vi "Dashboard Main.vi"() -> ()   [LabVIEW 2016]
uses:
  <vilib>/event_ctls.llb/eventvkey.ctl
  <vilib>/Rock Robotics/WPI/Dashboard/WPI_DashboardLogging Global.vi
  <vilib>/Utility/miscctls.llb/LVRowAndColumnTypeDef.ctl
  <vilib>/Rock Robotics/Network Tables/NT Read Numeric Array.vi
  <vilib>/Rock Robotics/Network Tables/NT Write Boolean.vi
panel:
  in  "Camera Settings Right":T1={"Frame Rate"=30, "Compression"=30, "Size"=1, "DB Camera Config"=FALSE} {"Frame Rate" scale=1.0..30.0; "Compression" scale=100.0..-1.0; "Size" items=["640x480", "320x240", "160x120"]}
  in  "Camera Name Right":string(combo)="No Camera Selection"
  out "Camera Info":cluster{"Mbps LED":bool, "Mbps":dbl, "fps":dbl} {"fps" format="%#.1g"; "Mbps" format="%#.1g"}
  in  "Camera Settings":T1={"Frame Rate"=30, "Compression"=30, "Size"=1, "DB Camera Config"=FALSE} {"Frame Rate" scale=1.0..30.0; "Compression" scale=100.0..-1.0; "Size" items=["640x480", "320x240", "160x120"]}
  in  "TCP":refnum<k5>
  in  "Rec Mode":enum32{"Stop", "Record", "Playback"}(radio)
  out "Robot IP":string
  out "Image Message":string="Timeout in Camera Communications"
  in  "Dashboard Tab":T2(tab)
  in  "Select Auto":string(combo)="Select Autonomous ..."
  out "NT Connection":bool
  out "MotorChart R":cluster{"Numeric":dbl, "Numeric":dbl}(graph)
  out "MotorChart L":cluster{"Numeric":dbl, "Numeric":dbl}(graph)
  out "MotorSliders R":cluster{"MotorSlide1":dbl, "MotorSlide2":dbl} {"MotorSlide2" scale=-1.0..1.0 scale format="%#_2e"; "MotorSlide1" scale=-1.0..1.0 scale format="%#_2e"}
  out "MotorSliders L":cluster{"MotorSlide1":dbl, "MotorSlide2":dbl} {"MotorSlide2" scale=-1.0..1.0 scale format="%#_2e"; "MotorSlide1" scale=-1.0..1.0 scale format="%#_2e"}
  out "Gyro":dbl(knob) scale=0.0..360.0
  out "JS1 Z":dbl(slide) scale=-1.0..1.0 scale format="%#_2e"
  out "JS1 Graph":cluster{"X":dbl, "Y":dbl}[](graph)
  out "JS1 Buttons":T3
  out "JS2 Z":dbl(slide) scale=-1.0..1.0 scale format="%#_2e"
  out "JS2 Graph":cluster{"X":dbl, "Y":dbl}[](graph)
  out "JS2 Buttons":T3
  out "Mode":T4(ring)=enum."Auto Disabled"
  in  "Overdrive Enabled?":bool
  in  "Trim":dbl(slide) scale=0.0..1.0
  out "Sonar":dbl
  out "Camera Image Right":T5(plugin-control)
  in  "DB/String 9":string
  in  "DB/String 8":string
  in  "DB/String 7":string
  in  "DB/String 6":string
  in  "DB/String 5":string
  in  "DB/String 4":string
  in  "DB/String 3":string
  in  "DB/String 2":string
  in  "DB/String 1":string
  in  "DB/String 0":string
  in  "DB/Slider 0":dbl(slide) scale=0.0..1.0
  in  "DB/Slider 1":dbl(slide) scale=0.0..5.0
  in  "DB/Slider 2":dbl(slide) scale=0.0..5.0
  in  "DB/Slider 3":dbl(slide) scale=0.0..5.0
  out "DB/LED 3":bool
  out "DB/LED 2":bool
  out "DB/LED 1":bool
  out "DB/LED 0":bool
  in  "DB/Button 3":bool
  in  "DB/Button 2":bool
  in  "DB/Button 1":bool
  in  "DB/Button 0":bool caption="New Name"
  in  "Scaling factor (V/in)":dbl=0.0098
  out "distance":dbl(slide)=125.0 scale=0.0..250.0 scale format="%3d"
  out "Z Acceleration":dbl
  out "Y Acceleration":dbl
  out "X Acceleration":dbl
  in  "Acc.Stop":bool
  in  "Test Slider":dbl(slide) scale=0.0..100.0 scale format="%#_3g"
  in  "On/Off":bool caption="Solenoid"
  in  "Test Name":u16(ring) items=["Select the test to run..."]
  in  "Test Tree":string(tree)
  in  "Motor":cluster{"Value":dbl, "Enable":bool} {"Value" scale=-1.0..1.0 scale format="%#_3g"}
  out "Progress":T6 {"Test Progress" scale=0.0..100.0}
  in  "Rev/Fwd":cluster{"Forward":bool, "Reverse":bool}
  in  "Test Ring":u16(ring) items=["Monochrome", "Color"]
  out "Cmd Status":string
  in  "Execute Command":bool
  in  "Command Params":string[][](table)
  in  "Command Selection":i32(listbox)
  in  "CheckList":i32(listbox)
  out "Tree":string(tree)
  out "Camera Image":T5(plugin-control)
  in  "Camera Name":string(combo)="No Camera Selection"
  # "HW"
  # "HW"
  # "Joysticks"
  # "Drive Motors"
  # "Front"
  # "Right"
  # "Left"
  # "Back"
  # "This tab is a great place for autonomous settings and robot-specific values.\nPlace controls and indicators inside this tab and match name to\nDashboard Variables on robot. You can also delete this comment."
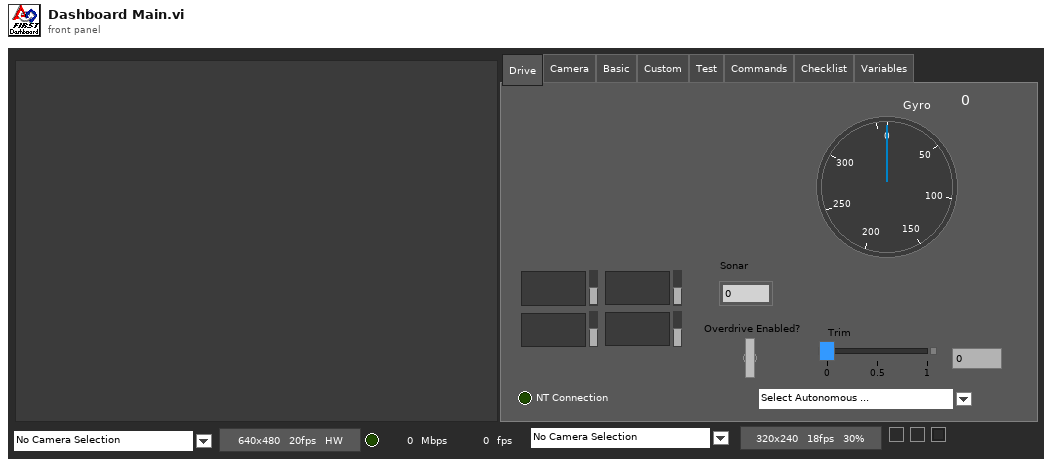
[diagram p1: front panel]
types:
  T1 = cluster{"Frame Rate":i32, "Compression":i32, "Size":u16, "DB Camera Config":bool}
  T2 = enum32{"Drive", "Camera", "Basic", "Custom", "Test", "Commands", "Checklist", "Variables"}
  T3 = cluster{bool, bool, bool, bool, bool, bool, bool, bool, bool, bool, bool, bool}
  T4 = enum8{"Tele-Op Disabled", "Tele-Op Enabled", "Auto Disabled", "Auto Enabled", "Test Disabled", "Test Enabled", "Disconnected", "No Code", "E-Stop"}
  T5 = typedef "IMAQ Image.ctl" = refnum<image>
  T6 = cluster{"Test Progress":u8, "Test Progress Text":string}
  T7 = typedef "Image Type" = u32
  T8 = cluster{"IDs":cluster{"RPC field ID":u16, "Unique ID":u16}, "String":string}
  T9 = enum32{"Drive", "Basic", "Custom", "Test", "Checklist", "Variables"}
  T10 = cluster{"Error Strings":string, "Disable Counts":cluster{u16, u16}, "Rail Faults":cluster{u16, u16, u16}, "Robot IP":string, "DB Mode":u8, "Event Info":cluster{"Name":string, "Type":u8, "Number":u16, "Replay":u8}}
  T11 = cluster{"Storage":cluster{"Disk Free":u64, "RAM Block":u32, "RAM free":u32}, "CPU Utilization":cluster{"CPU % ISR":sgl, "CPU % Time Crit":sgl, "CPU % Timed Str":sgl, "CPU % High":sgl, "CPU % Above":sgl, "CPU % Normal":sgl, "CPU % Low":sgl}, "CAN":cluster{"% Bus Utilization":sgl, "Bus Off Cnt":u32, "TX_FIFO Full Cnt":u32, "Receive Error Cnt":u8, "Transmit Error Cnt":u8}, "HID":cluster{"HID Outputs":u32, "Rumble Low":u16, "Rumble High":u16}[]}
  T12 = cluster{"Status bits":cluster{"Test Mode":bool, "Autonomous":bool, "Enabled":bool, "Code Start":bool, "Brownout":bool, "Reserved 2":bool, "Reserved 3":bool, "E-Stop":bool}, "Code Trace":cluster{"Disabled":bool, "TeleOp":bool, "Auto":bool, "Test":bool}, "Controller Type":enum16{"unknown", "cRIO", "roboRio"}, "Code?":enum16{"unknown", "noCode", "code"}, "Battery V":dbl}
  T13 = cluster{"Control Bits":cluster{"TestMode":bool, "Autonomous":bool, "Enabled":bool, "FMS Present":bool, bool, bool, bool, "E-Stop":bool}, "Team Station ":u8, "Countdown":sgl, "Joystick Values":cluster{"Axes":dbl[], "Buttons":bool[], "POVs":i16[]}[]}
  T14 = cluster{"Axes":dbl[], "Buttons":bool[], "POVs":i16[]}[]
  T15 = cluster{"Axes":dbl[], "Buttons":bool[], "POVs":i16[]}
  T16 = cluster{"Buttons[0]":bool, "Buttons[1]":bool, "Buttons[2]":bool, "Buttons[3]":bool, "Buttons[4]":bool, "Buttons[5]":bool, "Buttons[6]":bool, "Buttons[7]":bool, "Buttons[8]":bool, "Buttons[9]":bool, "Buttons[10]":bool, "Buttons[11]":bool}
  T17 = cluster{"Camera Image":refnum<vi>, "Dashboard Tab":refnum<vi>, void, "Rec Mode":refnum<vi>, "Test Slider":refnum<vi>, "On/Off ":refnum<vi>, "Test Ring":refnum<vi>, "Rev/Fwd":refnum<vi>, "Test Name":refnum<vi>, "Motor":refnum<vi>, "Progress":refnum<vi>, "CheckList":refnum<vi>, "Tree":refnum<vi>, "Test Tree":refnum<vi>, "Command Params":refnum<vi>, "Command Selection":refnum<vi>, "Execute Command":refnum<vi>, "Cmd Status":refnum<vi>, "Camera Settings":refnum<vi>, "Camera Name":refnum<vi>, "Camera Info":refnum<vi>, "Camera Settings Right":refnum<vi>, "Camera Name Right":refnum<vi>, "Camera Image Right":refnum<vi>}
  T18 = cluster{"Operation":enum16{"Update", "Clear"}, "Color Box":u32}[]
  T19 = typedef "eventvkey.ctl" = enum16{"ASCII", "Enter", "Return", "Shift", "Ctrl", "Alt", "Cmd", "Opt", "Caps", "NumLock", "Clear", "Break", "Up", "Down", "Left", "Right", "Insert", "Delete", "Home", "End", "PageUp", "PageDown", "Escape", "Help", "Pause", "ScrollLock", "F1", "F2", "F3", "F4", "F5", "F6", "F7", "F8", "F9", "F10", "F11", "F12", "F13", "F14", "F15", "F16", "F17", "F18", "F19", "F20", "F21", "F22", "F23", "F24", "Play", "VolumeUp", "VolumeDown", "Mute", "Two Byte Char"}
  T20 = cluster{"Image Size":bool, "Image Type":bool, "Pixel Value":bool, "ROI Information":bool, "Zoom Factor":bool}
  T21 = cluster{"Operation":enum16{"Update", "Clear"}, "Color Box":u32}
  T22 = typedef "LVRowAndColumnTypeDef.ctl" = cluster{"Row":i32, "Column":i32}
  T23 = cluster{"Shift":bool, "Ctrl":bool, "Alt":bool, "Cmd":bool, "Opt":bool}
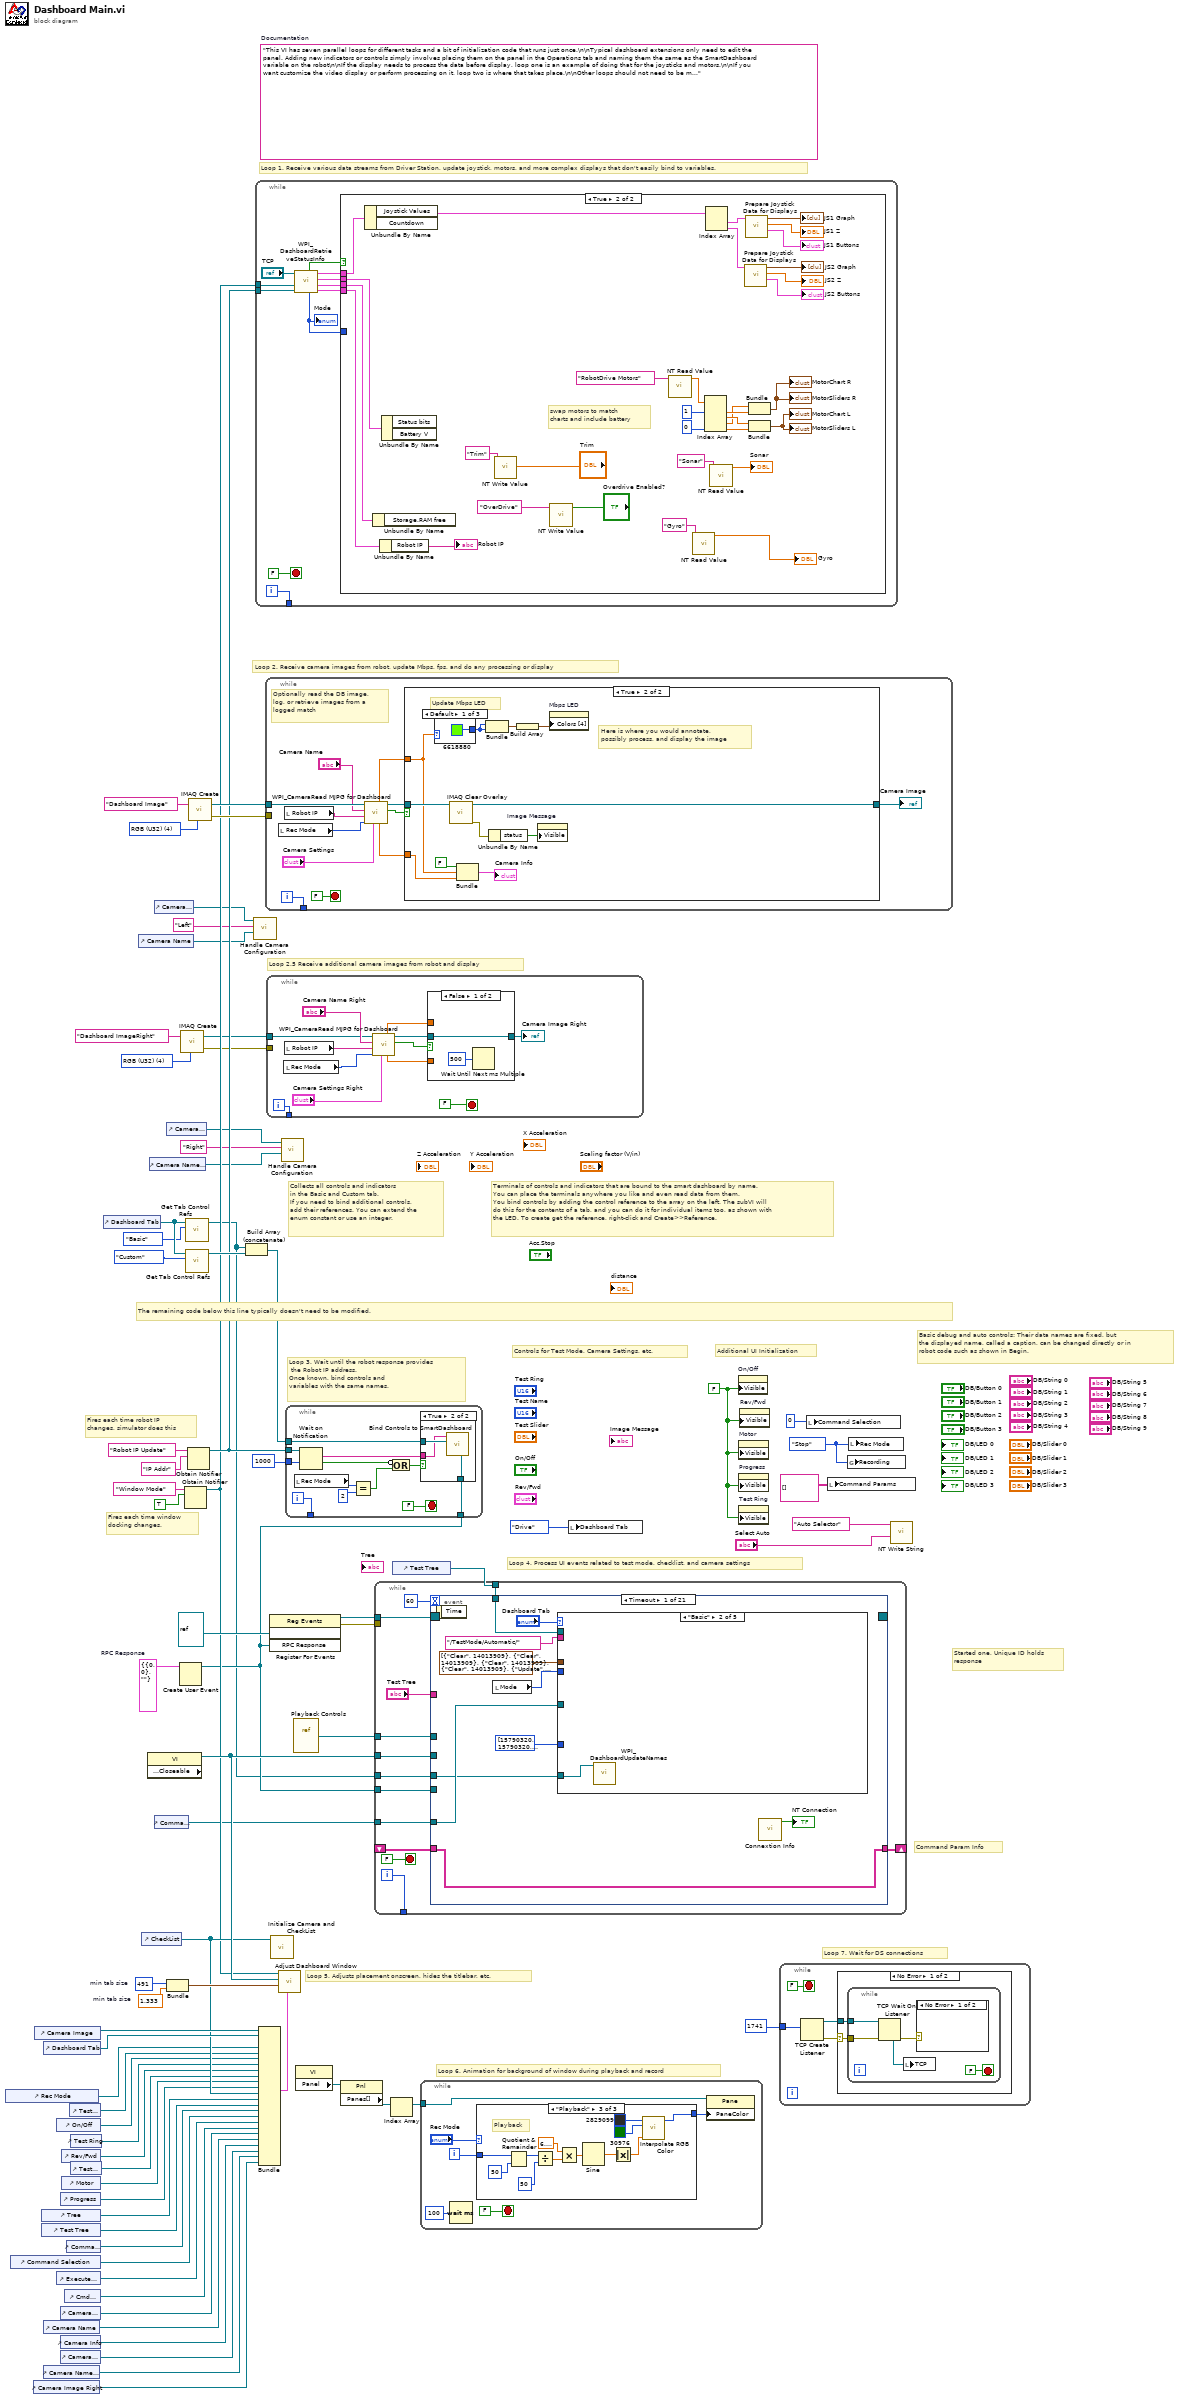
[diagram p0: block diagram]
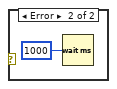
[diagram p3: hidden frame]
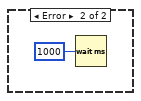
[diagram p4: hidden frame]
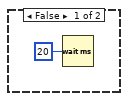
[diagram p5: hidden frame]
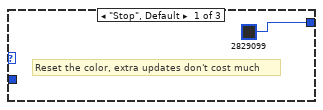
[diagram p6: hidden frame]
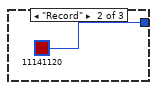
[diagram p7: hidden frame]
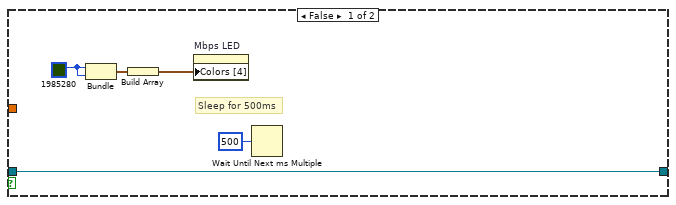
[diagram p9: hidden frame]
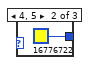
[diagram p10: hidden frame]
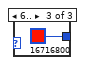
[diagram p11: hidden frame]
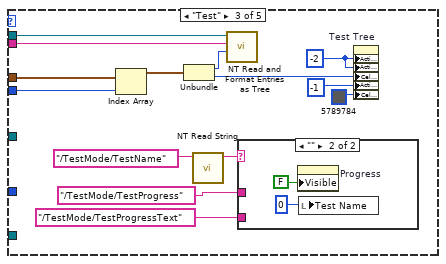
[diagram p13: hidden frame]
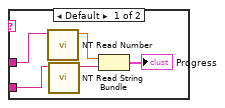
[diagram p14: hidden frame]
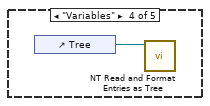
[diagram p15: hidden frame]
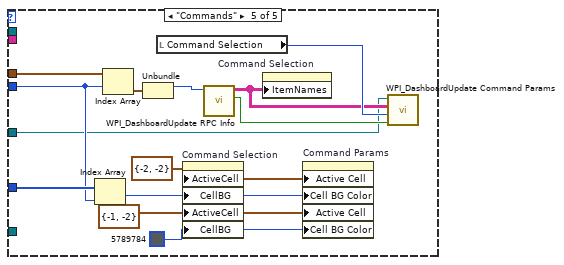
[diagram p16: hidden frame]
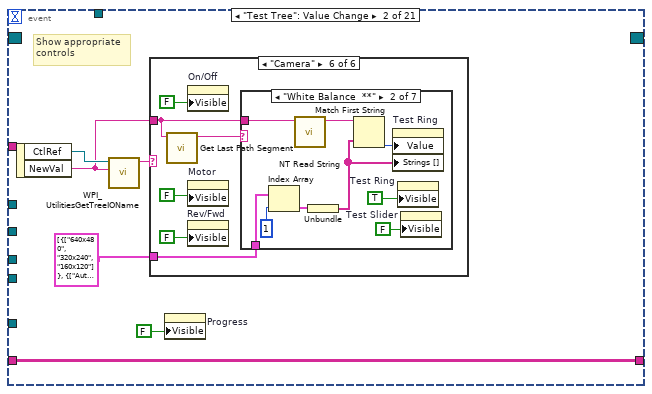
[diagram p17: hidden frame]
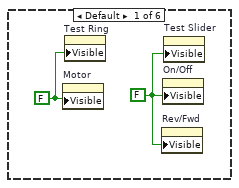
[diagram p18: hidden frame]
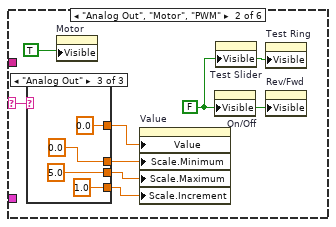
[diagram p19: hidden frame]
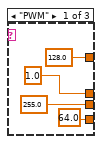
[diagram p20: hidden frame]
diagram:
  w11 = T7 4 items=["Grayscale (U8)", "Grayscale (I16)", "Grayscale (SGL)", "Complex (CSG)", "RGB (U32)", "HSL (U32)", "RGB (U64)"] ("Image Type")
  w27 = T8 {"IDs"={"RPC field ID"=0, "Unique ID"=0}, "String"=""}  # RPC Response
  w50 = 491  # min tab size
  w49 = 1.333  # min tab size
  w57 = enum32{"Stop", "Record", "Playback"}."Stop" ("Rec Mode")
  w34 = FALSE ("Visible")
  (unwired) "This VI has seven parallel loops for different tasks and a bit of initialization code that runs just once.\n\nTypical dashboard extensions only need to edit the panel. Adding new indicators or controls simply involves placing them on the panel in the Operations tab and naming them the same as the SmartDashboard variable on the robot\n\nIf the display needs to process the data before display, loop one is an example of doing that for the joysticks and motors.\n\nIf you want customize the video display or perform processing on it, loop two is where that takes place.\n\nOther loops should not need to be modified. They are pretty standard, and document the task they perform."  # Documentation
  w74 = T7 4 items=["Grayscale (U8)", "Grayscale (I16)", "Grayscale (SGL)", "Complex (CSG)", "RGB (U32)", "HSL (U32)", "RGB (U64)"] ("Image Type")
  # "Loop 2.5 Receive additional camera images from robot and display"
  # "Command Param Info"
  # "Started one, Unique ID holds\nresponse"
  # "Loop 7. Wait for DS connections"
  # "Basic debug and auto controls: Their data names are fixed, but\nthe displayed name, called a caption, can be changed directly or in\nrobot code such as shown in Begin."
  # "Controls for Test Mode, Camera Settings, etc."
  # "Additional UI Initialization"
  # "Loop 6. Animation for background of window during playback and record"
  # "Fires each time robot IP\nchanges, simulator does this"
  # "Fires each time window\ndocking changes."
  # "Collects all controls and indicators\nin the Basic and Custom tab.\nIf you need to bind additional controls,\nadd their references. You can extend the\nenum constant or use an integer."
  # "The remaining code below this line typically doesn't need to be modified."
  # "Loop 4. Process UI events related to test mode, checklist, and camera settings"
  # "Terminals of controls and indicators that are bound to the smart dashboard by name.\nYou can place the terminals anywhere you like and even read data from them.\nYou bind controls by adding the control reference to the array on the left. The subVI will\ndo this for the contents of a tab, and you can do it for individual items too, as shown with\nthe LED. To create get the reference, right-click and Create>>Reference."
  # "Loop 3. Wait until the robot response provides\n the Robot IP address.\nOnce known, bind controls and\nvariables with the same names."
  # "Loop 5. Adjusts placement onscreen, hides the titlebar, etc."
  # "Loop 1. Receive various data streams from Driver Station, update joystick, motors, and more complex displays that don't easily bind to variables."
  # "Loop 2. Receive camera images from robot, update Mbps, fps, and do any processing or display"
  n1 = control-ref of="Rec Mode"() -> (w40:refnum<vi>)
  n2 = control-ref of="Command Selection"() -> (w26:refnum<vi>)
  n3 = control-ref of="Camera Image Right"() -> (w2:refnum<vi>)
  n4 = control-ref of="Camera Image"() -> (w52:refnum<vi>)
  n5 = control-ref of="Tree"() -> (w44:refnum<vi>)
  n6 = control-ref of="Test Tree"() -> (w43:refnum<vi>)
  n7 = control-ref of="Dashboard Tab"() -> (w51:refnum<vi>)
  n8 = control-ref of="Camera Name"() -> (w17:refnum<vi>)
  n9 = control-ref of="Camera Name Right"() -> (w3:refnum<vi>)
  n10 = control-ref of="Execute Command"() -> (w28:refnum<vi>)
  n11 = control-ref of="On/Off"() -> (w38:refnum<vi>)
  n12 = control-ref of="Progress"() -> (w35:refnum<vi>)
  n13 = control-ref of="Camera Settings"() -> (w18:refnum<vi>)
  n14 = control-ref of="Camera Info"() -> (w16:refnum<vi>)
  n15 = control-ref of="Camera Settings Right"() -> (w4:refnum<vi>)
  n16 = control-ref of="Rev/Fwd"() -> (w36:refnum<vi>)
  n17 = control-ref of="Motor"() -> (w41:refnum<vi>)
  n18 = control-ref of="Cmd Status"() -> (w22:refnum<vi>)
  n19 = control-ref of="Command Params"() -> (w29:refnum<vi>)
  n20 = control-ref of="Test Slider"() -> (w39:refnum<vi>)
  n21 = control-ref of="Test Ring"() -> (w37:refnum<vi>)
  n22 = control-ref of="Test Name"() -> (w42:refnum<vi>)
  n23 = control-ref of="Dashboard Tab"() -> (w55:refnum<vi>)
  n24 = control-ref of="Camera Name"() -> (w19:refnum<vi>)
  n25 = control-ref of="CheckList"() -> (w45:refnum<vi>)
  n26 = property class="VI" props=["Front Panel.Closeable"]() -> (reference out=w56:refnum<vi>)  [unwired: 2 in, 2 out]
  n27 = control-ref of="Camera Name Right"() -> (w7:refnum<vi>)
  n28 = control-ref of="Camera Settings"() -> (w20:refnum<vi>)
  n29 = control-ref of="Command Params"() -> (w21:refnum<vi>)
  n30 = control-ref of="Camera Settings Right"() -> (w8:refnum<vi>)
  n31 = Bundle("min tab size"=w50, "min tab size"=w49) -> (w48:cluster{"min tab size":i32, "min tab size":dbl})  [unwired: 1 in]
  n32 = Create User Event(user event datatype=w27) -> (user event=w23:refnum<user-event>)  [unwired: 1 in, 1 out]
  n33 = call "IMAQ Create"("Image Name"="Dashboard ImageRight", "Image Type"=w11) -> ("New Image"=w10:T5, "error out"=w9:errorcluster)  [unwired: 2 in, 1 out]
  n34 = Obtain Notifier(name (unnamed)="Window Mode", notification data type=TRUE) -> (notifier out=w32:refnum<notifier>)  [unwired: 2 in, 2 out]
  n35 = call <vilib>:"Get Tab Control Refs.vi"("Page Index"=T9."Basic" ("Dashboard Tab"), "TabControl in"=w55) -> ("ControlsOnPage"=w15:refnum<vi>[])  [unwired: 9 in]
  n36 = call <vilib>:"Get Tab Control Refs.vi"("Page Index"=T9."Custom" ("Dashboard Tab"), "TabControl in"=w55) -> ("ControlsOnPage"=w54:refnum<vi>[])  [unwired: 9 in]
  n37 = Obtain Notifier(name (unnamed)="Robot IP Update", notification data type="IP Addr" ("name (unnamed)")) -> (notifier out=w33:refnum<notifier>)  [unwired: 2 in, 2 out]
  n38 = call "IMAQ Create"("Image Name"="Dashboard Image", "Image Type"=w74) -> ("New Image"=w72:T5, "error out"=w71:errorcluster)  [unwired: 2 in, 1 out]
  n39 = Build Array (concatenate)(w15, w54) -> (w53:refnum<vi>[])
  n40 = call "Handle Camera Configuration.vi"("CameraNameRef"=w19, "Camera File Name"="Left", "ClusterRef"=w20) -> ()  [unwired: 9 in]
  n41 = while {
    tunnel: [w84] -> _
    tunnel: w33 -> [w78]
    tunnel: w32 -> [w75]
    i -> [w84]
    stop <- FALSE stop-if-true
    n42 = call <vilib>:"WPI_DashboardRetrieveStatusInfo.vi"("Binding Refnum"=w78, "Window Mode Notifier"=w75, "TCP Cnx"="TCP") -> ("Power and Errors"=w79:T10, "Robot Metrics"=w82:T11, "Status Info"=w83:T12, "Control Info"=w80:T13, "Robot Mode"=w77:T4, "Process?"=w81:bool)  [unwired: 3 in]
    "Mode" <- w77
    n43 = case shown="True" w81 {
      tunnel: w83 -> [_ w118]
      tunnel: w82 -> [_ w117]
      tunnel: w80 -> [_ w116]
      tunnel: w79 -> [_ w115]
      tunnel: w77 -> [_ _]
      frame False {
        n44 = Wait (ms)(milliseconds to wait=u32 20) -> ()  [unwired: 1 out]
      }
      frame True {
        # "swap motors to match\ncharts and include battery"
        n45 = Unbundle By Name(w116) -> ("Joystick Values"=w106:T14)  [unwired: 1 out]
        n46 = Unbundle By Name(w117) -> ()  [unwired: 1 out]
        n47 = Unbundle By Name(w115) -> ("Robot IP"=→"Robot IP":string)
        n48 = Unbundle By Name(w118) -> ()  [unwired: 2 out]
        n49 = call-poly <vilib>:"NT Write Value.vi"("Numeric"="Trim", "Name"="Trim") -> ()  [unwired: 9 in, 1 out]
        n50 = call-poly <vilib>:"NT Write Value.vi"("Boolean"="Overdrive Enabled?", "Name"="OverDrive") -> ()  [unwired: 9 in, 1 out]
        n51 = call-poly <vilib>:"NT Read Value.vi"("Name"="RobotDrive Motors") -> ("Numeric Array"=w96:dbl[])  [unwired: 9 in, 1 out]
        n52 = call-poly <vilib>:"NT Read Value.vi"("Name"="Gyro") -> ("Numeric"=→"Gyro":dbl)  [unwired: 9 in, 1 out]
        n53 = Index Array(array=w96, index #1=1, index #4=0) -> (element #1=w110:dbl, element #2=w111:dbl, element #3=w109:dbl, element #4=w114:dbl)  [unwired: 2 in]
        n54 = Index Array(array=w106) -> (element #1=w105:T15, element #2=w101:T15)  [unwired: 2 in]
        n55 = call-poly <vilib>:"NT Read Value.vi"("Name"="Sonar") -> ("Numeric"=→"Sonar":dbl)  [unwired: 9 in, 1 out]
        n56 = call "Prepare Joystick Data for Displays.vi"("Joystick Values"=w101) -> ("Buttons"=→"JS2 Buttons":T16, "Z Axis"=→"JS2 Z":dbl, "Cartesian Data"=→"JS2 Graph":cluster{"X axis":dbl, "X axis":dbl}[])  [unwired: 8 in]
        n57 = call "Prepare Joystick Data for Displays.vi"("Joystick Values"=w105) -> ("Buttons"=→"JS1 Buttons":T16, "Z Axis"=→"JS1 Z":dbl, "Cartesian Data"=→"JS1 Graph":cluster{"X axis":dbl, "X axis":dbl}[])  [unwired: 8 in]
        n58 = Bundle("Numeric"=w109, "Numeric"=w110) -> (→"MotorChart R" →"MotorSliders R":cluster{"Numeric":dbl, "Numeric":dbl})  [unwired: 1 in]
        n59 = Bundle("Numeric"=w111, "Numeric"=w114) -> (→"MotorChart L" →"MotorSliders L":cluster{"Numeric":dbl, "Numeric":dbl})  [unwired: 1 in]
      }
    }
  }
  n60 = Bundle("Camera Image"=w52, "Dashboard Tab"=w51, "Rec Mode"=w40, "Test Slider"=w39, "On/Off"=w38, "Test Ring"=w37, "Rev/Fwd"=w36, "Test Name"=w42, "Motor"=w41, "Progress"=w35, "CheckList"=w45, "Tree"=w44, "Test Tree"=w43, "Command Params"=w29, "Command Selection"=w26, "Execute Command"=w28, "Cmd Status"=w22, "Camera Settings"=w18, "Camera Name"=w17, "Camera Info"=w16, "Camera Settings Right"=w4, "Camera Name Right"=w3, "Camera Image Right"=w2) -> (w1:T17)  [unwired: 2 in]
  n61 = while {
    tunnel: w72 -> [w128]
    tunnel: w71 -> [_]
    tunnel: [w129] -> _
    i -> [w129]
    stop <- FALSE stop-if-true
    # "Optionally read the DB image,\nlog, or retrieve images from a\nlogged match"
    n62 = local read "Rec Mode"() -> (w124:enum32{"Stop", "Record", "Playback"})
    n63 = local read "Robot IP"() -> (w123:string)
    n64 = call <vilib>:"WPI_CameraRead MJPG for Dashboard.vi"("Camera Settings"="Camera Settings", "Rec Mode"=w124, "Robot IP"=w123, "Camera Name"="Camera Name", "Refnum in"=w128) -> ("Active"=w126:bool, "Refnum out"=w127:T5, "FPS"=w125:dbl, "Bandwidth (Mbps)"=w122:dbl)  [unwired: 3 in]
    n65 = case shown="True" w126 {
      tunnel: w127 -> [w131 w142]
      tunnel: w122 -> [_ w139]
      tunnel: w125 -> [_ w140]
      tunnel: [w131 w136] -> w119
      frame False {
        w133 = u32 1985280 ("Color Box")
        # "Sleep for 500ms"
        n66 = Bundle("Color Box"=w133, "Color Box"=w133) -> (w134:cluster{"Color Box":u32, "Color Box":u32})  [unwired: 1 out]
        n67 = Build Array(w134) -> (w132:cluster{"Color Box":u32, "Color Box":u32}[])
        n68 = property on="Mbps LED" class="Bool (strict)"("Colors [4]"=w132) -> ()  [unwired: 2 in, 2 out]
        n69 = Wait Until Next ms Multiple(millisecond multiple=u32 500) -> ()  [unwired: 1 out]
      }
      frame True {
        # "Here is where you would annotate,\npossibly process, and display the image"
        # "Update Mbps LED"
        n70 = case shown="Default" w139 {
          tunnel: [u32 6618880 ("Color Box") u32 16776722 ("Color Box") u32 16716800 ("Color Box")] -> w143
          frame Default {
          }
          frame 4, 5 {
          }
          frame 6.. {
          }
        }
        n71 = call "IMAQ Clear Overlay"("Image"=w142) -> ("error out"=w145:errorcluster, "Image Out"=w136:T5)  [unwired: 2 in, 7 out]
        n72 = Bundle(FALSE, "Bandwidth (Mbps)"=w139, "FPS"=w140) -> (→"Camera Info":cluster{bool, "Bandwidth (Mbps)":dbl, "FPS":dbl})  [unwired: 1 in]
        n73 = Bundle("Color Box"=w143, "Color Box"=w143) -> (w144:cluster{"Color Box":u32, "Color Box":u32})  [unwired: 1 out]
        n74 = Unbundle By Name(w145) -> ("status"=w146:bool)
        n75 = Build Array(w144) -> (w141:cluster{"Color Box":u32, "Color Box":u32}[])
        n76 = property on="Image Message" class="Str"("Visible"=w146) -> ()  [unwired: 2 in, 2 out]
        n77 = property on="Mbps LED" class="Bool (strict)"("Colors [4]"=w141) -> ()  [unwired: 2 in, 2 out]
      }
    }
    "Camera Image" <- w119
  }
  n78 = while {
    tunnel: w10 -> [w160]
    tunnel: w9 -> [_]
    tunnel: [w154] -> _
    i -> [w154]
    stop <- FALSE stop-if-true
    n79 = local read "Rec Mode"() -> (w158:enum32{"Stop", "Record", "Playback"})
    n80 = local read "Robot IP"() -> (w159:string)
    n81 = call <vilib>:"WPI_CameraRead MJPG for Dashboard.vi"("Camera Settings"="Camera Settings Right", "Rec Mode"=w158, "Robot IP"=w159, "Camera Name"="Camera Name Right", "Refnum in"=w160) -> ("Active"=w153:bool, "Refnum out"=w156:T5, "FPS"=w151:dbl, "Bandwidth (Mbps)"=w152:dbl)  [unwired: 3 in]
    n82 = case shown="False" w153 {
      tunnel: w156 -> [w162 w164]
      tunnel: w152 -> [_ _]
      tunnel: w151 -> [_ _]
      tunnel: [w162 w164] -> w150
      frame False {
        n83 = Wait Until Next ms Multiple(millisecond multiple=u32 500) -> ()  [unwired: 1 out]
      }
      frame True {
      }
    }
    "Camera Image Right" <- w150
  }
  n84 = register-events(refnum<vi> refnum, w23) -> (reference out=w61:refnum<event-registration>, error out=w60:errorcluster)  [unwired: 2 in]
  n85 = call "Initialize Camera and CheckList.vi"("ListBox in"=w45) -> ()  [unwired: 11 in]
  n86 = call "Adjust Dashboard Window.vi"("Sizing Refnums"=w1, "Size Constraints"=w48, "VI"=w56, "WIn Mode"=w32) -> ()  [unwired: 8 in]
  n87 = call "Handle Camera Configuration.vi"("CameraNameRef"=w7, "Camera File Name"="Right", "ClusterRef"=w8) -> ()  [unwired: 9 in]
  n88 = while {
    tunnel: w53 -> [w176]
    tunnel: w33 -> [w174]
    tunnel: [w172] -> _
    tunnel: u32 1000 ("milliseconds to wait") -> [w171]
    tunnel: w23 -> [w165]
    i -> [w172]
    stop <- FALSE stop-if-true
    n89 = local read "Rec Mode"() -> (w167:enum32{"Stop", "Record", "Playback"})
    n90 = Wait on Notification(notifier=w174, timeout in ms (-1)=w171) -> (notification=w173:string, timed out?=w169:bool)  [unwired: 2 in, 2 out]
    n91 = Equal?(x=w167, y=u16 2 ("Rec Mode")) -> (x = y?=w168:bool)
    n92 = Compound Arithmetic op=OR(invert w169, w168) -> (w170:bool)
    n93 = case shown="True" w170 {
      tunnel: w176 -> [_ w179]
      tunnel: w173 -> [_ w178]
      tunnel: w165 -> [_ w177]
      frame False {
      }
      frame True {
        n94 = call <vilib>:"Bind Controls to SmartDashboard.vi"("RPC ref"=w177, "Bound Control Refs"=w179, "Server IP Address"=w178) -> ()  [unwired: 9 in]
      }
    }
  }
  n95 = vi-ref "Playback Controls.vi"() -> (w62:refnum<vi>)
  n96 = property class="VI"() -> ("Panel"=w64:refnum<vi>)  [unwired: 2 in, 2 out]
  n97 = property class="Pnl"(reference=w64) -> ("Panes[]"=w65:refnum<vi>[])  [unwired: 1 in, 2 out]
  n98 = Index Array(array=w65) -> (element=w63:refnum<vi>)  [unwired: 1 in]
  n99 = control-ref of="Test Tree"() -> (w66:refnum<vi>)
  n100 = while {
    tunnel: [w189] -> _
    tunnel: w66 -> [w188]
    tunnel: w62 -> [w187]
    tunnel: w61 -> [w186]
    tunnel: w60 -> [_]
    tunnel: w56 -> [w185]
    tunnel: w23 -> [w184]
    tunnel: w21 -> [w183]
    shift-right: [w182] -> _
    shift-left: _ -> [w181]
    tunnel: w15 -> [w180]
    i -> [w189]
    stop <- FALSE stop-if-true
    n101 = event shown="[0] Timeout" {
      selector: w186 -> [_ _ _ _ _ _ _ _ _ _ _ _ _ _ _ _ _ _ _ _ _]
      dyn-events: [_ _ _ _ _ _ _ _ _ _ _ _ _ _ _ _ w445 _ _ _ _] -> _
      timeout: u32 60 ("milliseconds to wait") -> [_ _ _ _ _ _ _ _ _ _ _ _ _ _ _ _ _ _ _ _ _]
      tunnel: w188 -> [w201 _ _ _ _ _ _ _ _ _ _ _ _ _ _ _ _ _ _ _ _]
      tunnel: "Test Tree" -> [_ _ _ _ _ _ _ _ _ _ _ w412 w420 w422 w426 w434 _ _ _ _ _]
      tunnel: w187 -> [_ _ _ _ _ _ _ _ _ _ _ _ _ _ _ _ w447 _ w465 _ _]
      tunnel: w185 -> [_ _ _ _ _ _ _ _ _ _ _ _ _ _ _ _ w443 _ _ _ _]
      tunnel: w184 -> [_ _ _ _ _ _ _ _ _ _ _ _ _ _ _ _ w439 _ _ _ _]
      tunnel: w183 -> [w196 _ _ _ _ _ w363 _ _ _ _ _ _ _ _ _ _ _ _ _ _]
      tunnel: [w195 w240 w342 w347 w356 w360 w361 w370 w380 w387 w399 w411 w418 w421 w425 w433 w438 w460 w462 w466 w477] -> w182
      tunnel: w181 -> [w195 w240 w342 w347 w356 w360 w361 _ _ w387 w399 w411 w418 w421 w425 w433 w438 w460 w462 w466 w477]
      tunnel: w180 -> [w193 _ _ _ _ _ _ _ _ _ _ _ _ _ _ _ _ _ _ _ _]
      event Timeout {
        n102 = event-data() -> ()  [unwired: 1 in, 1 out]
        n103 = local read "Mode"() -> (w198:T4)
        n104 = case shown="\"Basic\"" "Dashboard Tab" {
          tunnel: w201 -> [_ _ w217 _ _]
          tunnel: "/TestMode/Automatic/" ("Name Pattern") -> [_ _ w216 _ _]
          tunnel: T18 [{"Operation"=enum."Clear", "Color Box"=14013909}, {"Operation"=enum."Clear", "Color Box"=14013909}, {"Operation"=enum."Clear", "Color Box"=14013909}, {"Operation"=enum."Clear", "Color Box"=14013909}, {"Operation"=enum."Update", "Color Box"=14013909}, {"Operation"=enum."Update", "Color Box"=16777215}, {"Operation"=enum."Clear", "Color Box"=14013909}, {"Operation"=enum."Clear", "Color Box"=14013909}, {"Operation"=enum."Clear", "Color Box"=14013909}] -> [_ _ w209 _ w233]
          tunnel: w198 -> [_ _ w208 _ w232]
          tunnel: u32[] [15790320, 15790320, 15790320, 15790320, 16777215, 16777215, 15790320, 15790320, 15790320] -> [_ _ _ _ w238]
          tunnel: w196 -> [_ _ _ _ w226]
          tunnel: w193 -> [_ w203 _ _ _]
          frame "Custom", Default {
          }
          frame "Basic" {
            n105 = call <vilib>:"WPI_DashboardUpdateNames.vi"("Controls on Tab"=w203) -> ()  [unwired: 11 in]
          }
          frame "Test" {
            w215 = -2 ("Active Item:Row Number")
            n106 = Index Array(array=w209, index=w208) -> (element=w210:T21)
            n107 = Unbundle(w210) -> ("Operation"=w211:enum16{"Update", "Clear"}, "Color Box"=w212:u32)
            n108 = call <vilib>:"NT Read String.vi"("Name"="/TestMode/TestName") -> ("String"=w206:string)  [unwired: 9 in, 1 out]
            n109 = call <vilib>:"NT Read and Format Entries as Tree.vi"("Operation"=w211, "Name Pattern"=w216, "Tree Refnum"=w217) -> ()  [unwired: 7 in, 2 out]
            n110 = case shown="\"\"" w206 {
              tunnel: "/TestMode/TestProgress" ("Name") -> [w219 _]
              tunnel: "/TestMode/TestProgressText" ("Name") -> [w218 _]
              frame Default {
                n111 = call <vilib>:"NT Read Number.vi"("Name"=w219) -> ("Numeric"=w220:dbl)  [unwired: 9 in, 1 out]
                n112 = call <vilib>:"NT Read String.vi"("Name"=w218) -> ("String"=w221:string)  [unwired: 9 in, 1 out]
                n113 = Bundle("Numeric"=w220, "String"=w221) -> (→"Progress":cluster{"Numeric":dbl, "String":string})  [unwired: 1 in]
              }
              frame "" {
                n114 = property on="Progress" class="Clust (strict)"("Visible"=FALSE) -> ()  [unwired: 2 in, 2 out]
                n115 = local write "Test Name"(u16 0) -> ()
              }
            }
            n116 = property on="Test Tree" class="Tree (strict)"("Active Item Row Number"=w215, "ActiveColNum"=w215, "CellBG"=w212, "Active Item Row Number"=-1 ("Active Item:Row Number"), "CellBG"=u32 5789784 ("Color Box")) -> ()  [unwired: 2 in, 2 out]
          }
          frame "Variables" {
            n117 = control-ref of="Tree"() -> (w225:refnum<vi>)
            n118 = call <vilib>:"NT Read and Format Entries as Tree.vi"("Tree Refnum"=w225) -> ()  [unwired: 9 in, 2 out]
          }
          frame "Commands" {
            w234 = u32 5789784 ("Color Box")
            w235 = T22 {"Row"=-1, "Column"=-2} ("Active Cell:Active Cell")
            w237 = T22 {"Row"=-2, "Column"=-2} ("Active Cell:Active Cell")
            n119 = Index Array(array=w238, index=w232) -> (element=w236:u32)
            n120 = Index Array(array=w233, index=w232) -> (element=w231:T21)
            n121 = Unbundle(w231) -> ("Operation"=w230:enum16{"Update", "Clear"})  [unwired: 1 out]
            n122 = local read "Command Selection"() -> (w229:i32)
            n123 = property on="Command Selection" class="MCListbox (strict)"("ActiveCell"=w237, "CellBG"=w236, "ActiveCell"=w235, "CellBG"=w234) -> ()  [unwired: 2 in, 2 out]
            n124 = call <vilib>:"WPI_DashboardUpdate RPC Info.vi"("Operation"=w230) -> ("update"=w228:bool, "commands"=w227:string[][])  [unwired: 9 in]
            n125 = property on="Command Selection" class="MCListbox (strict)"("ItemNames"=w227) -> ()  [unwired: 2 in, 2 out]
            n126 = property on="Command Params" class="Tbl (strict)"("Active Cell"=w237, "Cell BG Color"=w236, "Active Cell"=w235, "Cell BG Color"=w234) -> ()  [unwired: 2 in, 2 out]
            n127 = call <vilib>:"WPI_DashboardUpdate Command Params.vi"("Update"=w228, "NewVal"=w229, "Commands"=w227, "Param Tbl"=w226) -> ()  [unwired: 7 in, 1 out]
          }
        }
        n128 = call <vilib>:"Connextion Info.vi"() -> ("Connected"=→"NT Connection":bool)  [unwired: 10 in, 1 out]
      }
      event "Test Tree": Value Change {
        # "Show appropriate\ncontrols"
        n129 = event-data() -> ("CtlRef"=w243:refnum<vi>, "NewVal"=w241:string)  [unwired: 1 in]
        n130 = call <vilib>:"WPI_UtilitiesGetTreeIOName.vi"("NewVal"=w241, "TreeControl in"=w243) -> ("I/O Name"=w244:string)  [unwired: 9 in]
        n131 = case shown="\"Camera\"" w244 {
          selector: w244 -> [_ w251 _ w273 w282 _]
          tunnel: w241 -> [_ _ w270 w272 _ w289]
          tunnel: cluster{string[]}[] [{["640x480", "320x240", "160x120"]}, {["Auto", "Fixed indoor", "Fixed outdoor 1", "Fixed outdoor 2", "Fixed fluorescent 1", "Fixed fluorescent 2", "Hold current"]}, {["Auto", "Flicker-free 50 Hz", "Flicker-free 60 Hz", "Hold current"]}, {["None", "Prioritize frame rate", "Prioritize image quality"]}, {["Monochrome", "Color"]}] -> [_ _ _ _ _ w288]
          frame Default {
            w246 = FALSE ("Visible")
            w245 = FALSE ("Visible")
            n132 = property on="Motor" class="Clust (strict)"("Visible"=w245) -> ()  [unwired: 2 in, 2 out]
            n133 = property on="Test Ring" class="Ring (strict)"("Visible"=w245) -> ()  [unwired: 2 in, 2 out]
            n134 = property on="Rev/Fwd" class="Clust (strict)"("Visible"=w246) -> ()  [unwired: 2 in, 2 out]
            n135 = property on="On/Off" class="Bool (strict)"("Visible"=w246) -> ()  [unwired: 2 in, 2 out]
            n136 = property on="Test Slider" class="Slide (strict)"("Visible"=w246) -> ()  [unwired: 2 in, 2 out]
          }
          frame "Analog Out", "Motor", "PWM" {
            w252 = FALSE ("Visible")
            n137 = case shown="\"Analog Out\"" w251 {
              tunnel: [1.0 ("Value") -1.0 ("Value") 0.0 ("Value")] -> w250
              tunnel: [255.0 ("Value") 1.0 ("Value") 5.0 ("Value")] -> w249
              tunnel: [128.0 ("Value") 0.0 ("Value") 0.0 ("Value")] -> w248
              tunnel: [64.0 ("Value") 0.5 ("Value") 1.0 ("Value")] -> w247
              frame "PWM" {
              }
              frame "Motor", Default {
              }
              frame "Analog Out" {
              }
            }
            n138 = property on="Motor" class="Clust (strict)"("Visible"=TRUE) -> ()  [unwired: 2 in, 2 out]
            n139 = property on="Value" class="Slide (strict)"("Value"=w248, "Scale.Minimum"=w250, "Scale.Maximum"=w249, "Scale.Increment"=w247) -> ()  [unwired: 2 in, 2 out]
            n140 = property on="On/Off" class="Bool (strict)"("Visible"=w252) -> ()  [unwired: 2 in, 2 out]
            n141 = property on="Test Slider" class="Slide (strict)"("Visible"=w252) -> ()  [unwired: 2 in, 2 out]
            n142 = property on="Test Ring" class="Ring (strict)"("Visible"=w252) -> ()  [unwired: 2 in, 2 out]
            n143 = property on="Rev/Fwd" class="Clust (strict)"("Visible"=w252) -> ()  [unwired: 2 in, 2 out]
          }
          frame "Servo" {
            w268 = FALSE ("Visible")
            n144 = call <vilib>:"NT Read Number.vi"("Name"=w270) -> ("Numeric"=w269:dbl)  [unwired: 9 in, 1 out]
            n145 = property on="Test Slider" class="Slide (strict)"("Visible"=TRUE, "Scale.Maximum"=170.0 ("Scale.Range:Maximum")) -> ()  [unwired: 2 in, 2 out]
            n146 = local write "Test Slider"(w269) -> ()
            n147 = property on="Motor" class="Clust (strict)"("Visible"=w268) -> ()  [unwired: 2 in, 2 out]
            n148 = property on="Rev/Fwd" class="Clust (strict)"("Visible"=w268) -> ()  [unwired: 2 in, 2 out]
            n149 = property on="On/Off" class="Bool (strict)"("Visible"=w268) -> ()  [unwired: 2 in, 2 out]
            n150 = property on="Test Ring" class="Ring (strict)"("Visible"=w268) -> ()  [unwired: 2 in, 2 out]
          }
          frame "Relay", "Solenoid" {
            w271 = FALSE ("Visible")
            n151 = property on="Motor" class="Clust (strict)"("Visible"=w271) -> ()  [unwired: 2 in, 2 out]
            n152 = property on="Test Slider" class="Slide (strict)"("Visible"=w271) -> ()  [unwired: 2 in, 2 out]
            n153 = Search and Replace String(input string=w272, search string="/Value  **", replace string="/Direction") -> (result string=w278:string)  [unwired: 5 in, 3 out]
            n154 = property on="Test Ring" class="Ring (strict)"("Visible"=w271) -> ()  [unwired: 2 in, 2 out]
            n155 = call <vilib>:"NT Read String.vi"("Name"=w278) -> ("String"=w276:string)  [unwired: 9 in, 1 out]
            n156 = Equal?(x="Both directions", y=w276) -> (x = y?=w274:bool)
            n157 = Not(x=w274) -> (.not. x?=w275:bool)
            n158 = property on="Rev/Fwd" class="Clust (strict)"("Visible"=w274) -> ()  [unwired: 2 in, 2 out]
            n159 = property on="On/Off" class="Bool (strict)"("Visible"=w275, "Caption.Text"=w273) -> ()  [unwired: 2 in, 2 out]
          }
          frame "Compressor", "Digital Out" {
            w281 = FALSE ("Visible")
            # "Get direction and finish"
            n160 = property on="Motor" class="Clust (strict)"("Visible"=w281) -> ()  [unwired: 2 in, 2 out]
            n161 = property on="Test Slider" class="Slide (strict)"("Visible"=w281) -> ()  [unwired: 2 in, 2 out]
            n162 = property on="Test Ring" class="Ring (strict)"("Visible"=w281) -> ()  [unwired: 2 in, 2 out]
            n163 = property on="On/Off" class="Bool (strict)"("Visible"=TRUE, "Caption.Text"=w282) -> ()  [unwired: 2 in, 2 out]
            n164 = property on="Rev/Fwd" class="Clust (strict)"("Visible"=FALSE) -> ()  [unwired: 2 in, 2 out]
          }
          frame "Camera" {
            n165 = call <vilib>:"Get Last Path Segment.vi"("String in"=w289) -> ("String out"=w290:string)  [unwired: 10 in]
            n166 = property on="On/Off" class="Bool (strict)"("Visible"=FALSE) -> ()  [unwired: 2 in, 2 out]
            n167 = property on="Motor" class="Clust (strict)"("Visible"=FALSE) -> ()  [unwired: 2 in, 2 out]
            n168 = property on="Rev/Fwd" class="Clust (strict)"("Visible"=FALSE) -> ()  [unwired: 2 in, 2 out]
            n169 = case shown="\"White Balance  **\"" w290 {
              tunnel: w289 -> [w296 w305 w314 w323 w332 _ w338]
              tunnel: w288 -> [w294 w302 w311 w320 w329 _ _]
              frame "Size  **" {
                n170 = Index Array(array=w294) -> (element=w293:cluster{string[]})  [unwired: 1 in]
                n171 = call <vilib>:"NT Read String.vi"("Name"=w296) -> ("String"=w295:string)  [unwired: 9 in, 1 out]
                n172 = Unbundle(w293) -> (w291:string[])
                n173 = Match First String(2:w291, 3:w295) -> (0:w292:i32)  [unwired: 1 out]
                n174 = property on="Test Ring" class="Ring (strict)"("Value"=w292, "Strings []"=w291) -> ()  [unwired: 2 in, 2 out]
                n175 = property on="Test Ring" class="Ring (strict)"("Visible"=TRUE) -> ()  [unwired: 2 in, 2 out]
                n176 = property on="Test Slider" class="Slide (strict)"("Visible"=FALSE) -> ()  [unwired: 2 in, 2 out]
              }
              frame "White Balance  **" {
                n177 = Index Array(array=w302, index=1) -> (element=w303:cluster{string[]})
                n178 = call <vilib>:"NT Read String.vi"("Name"=w305) -> ("String"=w304:string)  [unwired: 9 in, 1 out]
                n179 = Unbundle(w303) -> (w300:string[])
                n180 = Match First String(2:w300, 3:w304) -> (0:w299:i32)  [unwired: 1 out]
                n181 = property on="Test Ring" class="Ring (strict)"("Value"=w299, "Strings []"=w300) -> ()  [unwired: 2 in, 2 out]
                n182 = property on="Test Ring" class="Ring (strict)"("Visible"=TRUE) -> ()  [unwired: 2 in, 2 out]
                n183 = property on="Test Slider" class="Slide (strict)"("Visible"=FALSE) -> ()  [unwired: 2 in, 2 out]
              }
              frame "Exposure  **" {
                n184 = Index Array(array=w311, index=2) -> (element=w312:cluster{string[]})
                n185 = call <vilib>:"NT Read String.vi"("Name"=w314) -> ("String"=w313:string)  [unwired: 9 in, 1 out]
                n186 = Unbundle(w312) -> (w308:string[])
                n187 = Match First String(2:w308, 3:w313) -> (0:w309:i32)  [unwired: 1 out]
                n188 = property on="Test Ring" class="Ring (strict)"("Value"=w309, "Strings []"=w308) -> ()  [unwired: 2 in, 2 out]
                n189 = property on="Test Ring" class="Ring (strict)"("Visible"=TRUE) -> ()  [unwired: 2 in, 2 out]
                n190 = property on="Test Slider" class="Slide (strict)"("Visible"=FALSE) -> ()  [unwired: 2 in, 2 out]
              }
              frame "Exposure Priority  **" {
                n191 = Index Array(array=w320, index=3) -> (element=w321:cluster{string[]})
                n192 = call <vilib>:"NT Read String.vi"("Name"=w323) -> ("String"=w322:string)  [unwired: 9 in, 1 out]
                n193 = Unbundle(w321) -> (w317:string[])
                n194 = Match First String(2:w317, 3:w322) -> (0:w318:i32)  [unwired: 1 out]
                n195 = property on="Test Ring" class="Ring (strict)"("Value"=w318, "Strings []"=w317) -> ()  [unwired: 2 in, 2 out]
                n196 = property on="Test Ring" class="Ring (strict)"("Visible"=TRUE) -> ()  [unwired: 2 in, 2 out]
                n197 = property on="Test Slider" class="Slide (strict)"("Visible"=FALSE) -> ()  [unwired: 2 in, 2 out]
              }
              frame "Color Enable  **" {
                n198 = Index Array(array=w329, index=4) -> (element=w330:cluster{string[]})
                n199 = call <vilib>:"NT Read String.vi"("Name"=w332) -> ("String"=w331:string)  [unwired: 9 in, 1 out]
                n200 = Unbundle(w330) -> (w326:string[])
                n201 = Match First String(2:w326, 3:w331) -> (0:w327:i32)  [unwired: 1 out]
                n202 = property on="Test Ring" class="Ring (strict)"("Value"=w327, "Strings []"=w326) -> ()  [unwired: 2 in, 2 out]
                n203 = property on="Test Ring" class="Ring (strict)"("Visible"=TRUE) -> ()  [unwired: 2 in, 2 out]
                n204 = property on="Test Slider" class="Slide (strict)"("Visible"=FALSE) -> ()  [unwired: 2 in, 2 out]
              }
              frame Default {
                n205 = property on="Test Ring" class="Ring (strict)"("Visible"=FALSE) -> ()  [unwired: 2 in, 2 out]
                n206 = property on="Test Slider" class="Slide (strict)"("Visible"=FALSE) -> ()  [unwired: 2 in, 2 out]
              }
              frame "Brightness  **", "Color Level  **", "Compression  **", "FPS  **", "Sharpness  **" {
                n207 = call <vilib>:"NT Read Number.vi"("Name"=w338) -> ("Numeric"=w337:dbl)  [unwired: 9 in, 1 out]
                n208 = local write "Test Slider"(w337) -> ()
                n209 = property on="Test Slider" class="Slide (strict)"("Visible"=TRUE, "Scale.Maximum"=100.0 ("Scale.Range:Maximum")) -> ()  [unwired: 2 in, 2 out]
                n210 = property on="Test Ring" class="Ring (strict)"("Visible"=FALSE) -> ()  [unwired: 2 in, 2 out]
              }
            }
          }
        }
        n211 = property on="Progress" class="Clust (strict)"("Visible"=FALSE) -> ()  [unwired: 2 in, 2 out]
      }
      event "Test Name": Mouse Enter {
        # "Populate the ring with the list of tests"
        n212 = event-data() -> ()  [unwired: 1 in, 1 out]
        n213 = call <vilib>:"NT Read String Array.vi"("Name"="/TestMode/TestList") -> ("String Array"=w346:string[])  [unwired: 9 in, 1 out]
        n214 = Build Array (concatenate)("Select the test to run...", w346) -> (w345:string[])
        n215 = property on="Test Name" class="Ring (strict)"("Strings []"=w345) -> ()  [unwired: 2 in, 2 out]
      }
      event "Test Name": Value Change {
        w348 = FALSE ("Visible")
        # "Tell the robot the test name to run"
        n216 = event-data() -> ("NewVal"=w352:u16)  [unwired: 1 in]
        n217 = property on="Test Name" class="Ring (strict)"() -> ("Strings []"=w353:string[])  [unwired: 2 in, 2 out]
        n218 = local write "Progress"(T6 {"Test Progress"=0, "Test Progress Text"=""} ("Progress")) -> ()
        n219 = Index Array(array=w353, index=w352) -> (element=w351:string)
        n220 = call <vilib>:"NT Write String.vi"("String"=w351, "Name"="/TestMode/TestName") -> ()  [unwired: 9 in, 1 out]
        n221 = property on="Progress" class="Clust (strict)"("Visible"=TRUE) -> ()  [unwired: 2 in, 2 out]
        n222 = property on="Motor" class="Clust (strict)"("Visible"=w348) -> ()  [unwired: 2 in, 2 out]
        n223 = property on="Test Slider" class="Slide (strict)"("Visible"=w348) -> ()  [unwired: 2 in, 2 out]
        n224 = property on="On/Off" class="Bool (strict)"("Visible"=w348) -> ()  [unwired: 2 in, 2 out]
        n225 = property on="Rev/Fwd" class="Clust (strict)"("Visible"=w348) -> ()  [unwired: 2 in, 2 out]
        n226 = property on="Test Ring" class="Ring (strict)"("Visible"=w348) -> ()  [unwired: 2 in, 2 out]
      }
      event "Select Auto": Mouse Enter {
        # "Populate the combo box with the list of autonomous options"
        n227 = event-data() -> ()  [unwired: 1 in, 1 out]
        n228 = call <vilib>:"NT Read String Array.vi"("Name"="Auto List") -> ("String Array"=w355:string[])  [unwired: 9 in, 1 out]
        n229 = property on="Select Auto" class="CmbBox"("Strings[]"=w355) -> ()  [unwired: 2 in, 2 out]
      }
      event "Select Auto": Value Change {
        # "User modified the Auto Selection. Write to NT variable so robot knows."
        n230 = event-data() -> ("NewVal"=w358:string)  [unwired: 1 in]
        n231 = call <vilib>:"NT Write String.vi"("String"=w358, "Name"="Auto Selector") -> ()  [unwired: 9 in, 1 out]
      }
      event "Command Selection": Value Change {
        # "Get the params and show in table"
        n232 = event-data() -> ("NewVal"=w364:i32)  [unwired: 1 in]
        n233 = property on="Command Selection" class="MCListbox (strict)"() -> ("ItemNames"=w362:string[][])  [unwired: 2 in, 2 out]
        n234 = call <vilib>:"WPI_DashboardUpdate Command Params.vi"("NewVal"=w364, "Commands"=w362, "Param Tbl"=w363) -> ()  [unwired: 8 in, 1 out]
      }
      event "Execute Command": Value Change {
        # "Started one, Unique ID holds\nresponse"
        n235 = event-data() -> ()  [unwired: 1 in, 1 out]
        n236 = property on="Command Selection" class="MCListbox (strict)"() -> ("ItemNames"=w375:string[][])  [unwired: 2 in, 2 out]
        n237 = Index Array(array=w375, index (row)="Command Selection", index (col)=0) -> (element=w373:string)
        n238 = call <vilib>:"Invoke Commands.vi"("Command Params"="Command Params", "Function Name"=w373) -> ("Params"=w369:u8, "Started"=w368:bool)  [unwired: 7 in, 1 out]
        n239 = Array Subset(array="Command Params", length (row)=w369) -> (w370:string[][])  [unwired: 3 in]
        n240 = Select(t="Executing" ("Cmd Status"), s=w368, f="" ("Cmd Status")) -> (s? t:f=→"Cmd Status":string)
      }
      event "Command Selection": Double Click {
        n241 = event-data() -> ("Row"=w383:i32)  [unwired: 1 in]
        n242 = property on="Command Selection" class="MCListbox (strict)"() -> ("ItemNames"=w386:string[][])  [unwired: 2 in, 2 out]
        n243 = local read "Command Params"() -> (w382:string[][])
        n244 = Index Array(array=w386, index (row)=w383, index (col)=0) -> (element=w384:string)
        n245 = call <vilib>:"Invoke Commands.vi"("Command Params"=w382, "Function Name"=w384) -> ("Params"=w381:u8, "Started"=w376:bool)  [unwired: 7 in, 1 out]
        n246 = Array Subset(array=w382, length (row)=w381) -> (w380:string[][])  [unwired: 3 in]
        n247 = Select(t="Executing" ("Cmd Status"), s=w376, f="" ("Cmd Status")) -> (s? t:f=w377:string)
        n248 = local write "Cmd Status"(w377) -> ()
      }
      event "CheckList": Double Click {
        # "Shift clears all"
        # "Update symbols on the listbox"
        n249 = event-data() -> ("PlatMods.Shift"=w388:bool, "Row"=w390:i32)  [unwired: 1 in]
        n250 = case shown="True" w388 {
          tunnel: w390 -> [w394 _]
          tunnel: 1 -> [w393 _]
          frame False {
            n251 = property on="CheckList" class="LstBox (strict)"() -> ("Item Symbols"=w392:i32[])  [unwired: 2 in, 2 out]
            n252 = Replace Array Subset(array=w392, new element=w393, index=w394) -> (w391:i32[])
            n253 = property on="CheckList" class="LstBox (strict)"("Item Symbols"=w391) -> ()  [unwired: 2 in, 2 out]
          }
          frame True {
            w395 = 0 ("Top Row")
            n254 = property on="CheckList" class="LstBox (strict)"() -> ("Number of Rows"=w397:u32)  [unwired: 2 in, 2 out]
            n255 = Initialize Array(0, w397) -> (w396:i32[])
            n256 = property on="CheckList" class="LstBox (strict)"("Top Row"=w395, "Value"=w395, "Item Symbols"=w396) -> ()  [unwired: 2 in, 2 out]
          }
        }
      }
      event "CheckList": Key Down {
        # "Update symbols on the listbox\nLeft and right keys check and uncheck"
        n257 = event-data() -> ("VKey"=w401:T19)  [unwired: 1 in]
        n258 = case shown="\"Left\", \"Right\"" w401 {
          selector: w401 -> [w406 _]
          tunnel: eventvkey."Left" ("VKey") -> [w404 _]
          frame "Left", "Right" {
            n259 = Equal?(x=w404, y=w406) -> (x = y?=w405:bool)
            n260 = Select(t=0, s=w405, f=1) -> (s? t:f=w407:i32)
            n261 = property on="CheckList" class="LstBox (strict)"() -> ("Item Symbols"=w410:i32[])  [unwired: 2 in, 2 out]
            n262 = Replace Array Subset(array=w410, new element=w407, index="CheckList") -> (w409:i32[])
            n263 = property on="CheckList" class="LstBox (strict)"("Item Symbols"=w409) -> ()  [unwired: 2 in, 2 out]
          }
          frame Default {
          }
        }
      }
      event "Motor.Enable": Value Change {
        # "When the test mode otor enable helper is set, update that\ntree row item's value"
        n264 = event-data() -> ("NewVal"=w416:bool)  [unwired: 1 in]
        n265 = Unbundle("Motor") -> ("Value"=w415:dbl)  [unwired: 1 out]
        n266 = Select(t=w415, s=w416, f=0.0) -> (s? t:f=w413:dbl)
        n267 = call <vilib>:"NT Write Number.vi"("Numeric"=w413, "Name"=w412) -> ()  [unwired: 9 in, 1 out]
      }
      event "Test Slider": Value Change {
        # "When the test mode slider helper is set, update that\ntree row item's value"
        n268 = event-data() -> ("NewVal"=w419:dbl)  [unwired: 1 in]
        n269 = call <vilib>:"NT Write Number.vi"("Numeric"=w419, "Name"=w420) -> ()  [unwired: 9 in, 1 out]
      }
      event "On/Off": Value Change {
        # "When the test mode on/off helper value is set, update that\ntree row item's value"
        n270 = event-data() -> ("NewVal"=w424:bool)  [unwired: 1 in]
        n271 = Boolean To (0,1)(Boolean=w424) -> (0, 1=w423:i16)
        n272 = call <vilib>:"NT Write Number.vi"("Numeric"=w423, "Name"=w422) -> ()  [unwired: 9 in, 1 out]
      }
      event "Rev/Fwd": Value Change {
        # "When the test mode helper value for relays is set, update that\ntree row item's value"
        n273 = event-data() -> ("NewVal.Forward"=w432:bool, "NewVal.Reverse"=w431:bool)  [unwired: 1 in]
        n274 = Boolean To (0,1)(Boolean=w432) -> (0, 1=w428:i16)
        n275 = Boolean To (0,1)(Boolean=w431) -> (0, 1=w430:i16)
        n276 = Negate(x=w430) -> (-x=w429:i16)
        n277 = Add(x=w428, y=w429) -> (x+y=w427:i16)
        n278 = call <vilib>:"NT Write Number.vi"("Numeric"=w427, "Name"=w426) -> ()  [unwired: 9 in, 1 out]
      }
      event "Test Ring": Value Change {
        # "When a test mode helper value is selected from the ring,\nset the tree item's variable to the string value"
        n279 = event-data() -> ("NewVal"=w436:u16)  [unwired: 1 in]
        n280 = property on="Test Ring" class="Ring (strict)"() -> ("Strings []"=w437:string[])  [unwired: 2 in, 2 out]
        n281 = Index Array(array=w437, index=w436) -> (element=w435:string)
        n282 = call <vilib>:"NT Write String.vi"("String"=w435, "Name"=w434) -> ()  [unwired: 9 in, 1 out]
      }
      event "Rec Mode": Value Change {
        # "Update globals for recording mode and path to read log from.\nClear when logging and let NetworkTables set path for vision to\nuse."
        n283 = event-data() -> ("NewVal"=w448:enum32{"Stop", "Record", "Playback"})  [unwired: 1 in]
        n284 = global write "WPI_DashboardLogging Global.vi" "Logging Filename"(path "") -> ()
        n285 = global write "WPI_DashboardLogging Global.vi" "Recording"(w448) -> ()
        n286 = case shown="\"Playback\"" w448 {
          tunnel: w447 -> [_ w450 w459]
          tunnel: [_ _ w458] -> w445
          tunnel: [_ _ w457] -> _
          tunnel: w443 -> [_ _ w455]
          tunnel: cluster{i32, i32} {-250, 170} -> [_ _ w454]
          tunnel: [_ _ T20 {"Image Size"=TRUE, "Image Type"=TRUE, "Pixel Value"=TRUE, "ROI Information"=TRUE, "Zoom Factor"=FALSE} ("Image Information Shown:All Elements")] -> w441
          tunnel: [_ _ TRUE ("Zoom Factor")] -> w440
          tunnel: w439 -> [_ _ w451]
          frame Default {
          }
          frame "Stop", "Record" {
            # "Place Window too"
            n287 = invoke class="VI" method="FP.Close"(reference=w450) -> (reference out=w449:refnum<vi>)  [unwired: 2 in, 2 out]
            n288 = invoke class="VI" method="Abort VI"(reference=w449) -> ()  [unwired: 2 in, 3 out]
          }
          frame "Playback" {
            n289 = call "Open Playback Panel.vi"("Offset"=w454, "DB VI Ref"=w455, "Playback in"=w459) -> ("Playback out"=w456:refnum<vi>)  [unwired: 8 in]
            n290 = register-events(w456, w451) -> (reference out=w458:refnum<event-registration>, error out=w457:errorcluster)  [unwired: 2 in]
          }
        }
        n291 = property on="Camera Image" class="ImageControl"("Image Information Shown"=w441, "Image Information Visible"=w440) -> ()  [unwired: 2 in, 2 out]
        n292 = call <vilib>:"WPI_DashboardNT Log FieldName Cache.vi"("Operation"=enum16{"Lookup/Add", "Index", "Clear"}."Clear") -> ()  [unwired: 8 in, 3 out]
      }
      event Panel Close {
        w461 = enum32{"Stop", "Record", "Playback"}."Stop" ("Rec Mode")
        # "Playback window has been closed, abort"
        n293 = event-data() -> ()  [unwired: 1 in, 4 out]
        n294 = local write "Rec Mode"(w461) -> ()
        n295 = global write "WPI_DashboardLogging Global.vi" "Recording"(w461) -> ()
      }
      event Panel Close {
        # "Abort playback window and ourself"
        n296 = event-data() -> ()  [unwired: 1 in, 4 out]
        n297 = invoke class="VI" method="FP.Close"(reference=w465) -> (reference out=w464:refnum<vi>)  [unwired: 2 in, 2 out]
        n298 = invoke class="VI" method="Abort VI"(reference=w464) -> (error out=w463:errorcluster)  [unwired: 2 in, 2 out]
        n299 = invoke class="VI" method="Abort VI"(error in=w463) -> ()  [unwired: 2 in, 3 out]
      }
      event User Event {
        n300 = event-data() -> ("IDs"=w472:cluster{"RPC field ID":u16, "Unique ID":u16}, "String"=w471:string)  [unwired: 1 in]
        n301 = Bundle("IDs"=w472, "String"=w471) -> (w470:T8)  [unwired: 1 in]
        n302 = call <vilib>:"Retrieve RPC Response.vi"("RPC Response"=w470) -> ("Output"=w468:string[][])  [unwired: 10 in]
        n303 = Build Array (concatenate)(w466, w468) -> (w467:string[][])
        n304 = local write "Command Params"(w467) -> ()
        n305 = local write "Cmd Status"("" ("Cmd Status")) -> ()
      }
      event "Tree": Double Click {
        n306 = event-data() -> ("PlatMods"=w476:T23, "Tag"=w475:string)  [unwired: 1 in]
        n307 = Unbundle(w476) -> ("Shift"=w474:bool)  [unwired: 4 out]
        n308 = Not(x=w474) -> (.not. x?=w473:bool)
        n309 = call <vilib>:"NT Update Persistence.vi"("Persistence"=w473, "Name"=w475) -> ()  [unwired: 9 in, 1 out]
      }
    }
  }
  n310 = while {
    tunnel: w63 -> [w479]
    i -> [w482]
    stop <- FALSE stop-if-true
    n311 = Wait (ms)(milliseconds to wait=u32 100) -> ()  [unwired: 1 out]
    n312 = case shown="\"Playback\"" "Rec Mode" {
      tunnel: w482 -> [_ _ w497]
      tunnel: [u32 2829099 ("Base Color") u32 11141120 ("Target Color") w486] -> w478
      frame "Stop", Default {
        # "Reset the color, extra updates don't cost much"
      }
      frame "Record" {
      }
      frame "Playback" {
        # "Playback"
        n313 = Quotient & Remainder(x=w497, y=u32 50 ("milliseconds to wait")) -> (x-y*floor(x/y)=w493:u32)  [unwired: 1 out]
        n314 = Divide(x=w493, y=u32 50 ("milliseconds to wait")) -> (x/y=w490:dbl)
        n315 = Multiply(x=6.283185307179586, y=w490) -> (x*y=w495:dbl)
        n316 = Sine(x=w495) -> (sin(x)=w494:dbl)
        n317 = Absolute Value(x=w494) -> (abs(x)=w487:dbl)
        n318 = call "Interpolate RGB Color.vi"("Proportion"=w487, "Target Color"=u32 30976, "Base Color"=u32 2829099) -> ("Result Color"=w486:u32)  [unwired: 8 in]
      }
    }
    n319 = property class="Pane"(reference=w479, "PaneColor"=w478) -> ()  [unwired: 1 in, 2 out]
  }
  n320 = local write "Dashboard Tab"(T2."Drive" ("Dashboard Tab")) -> ()
  n321 = property on="On/Off" class="Bool (strict)"("Visible"=w34) -> ()  [unwired: 2 in, 2 out]
  n322 = property on="Motor" class="Clust (strict)"("Visible"=w34) -> ()  [unwired: 2 in, 2 out]
  n323 = property on="Progress" class="Clust (strict)"("Visible"=w34) -> ()  [unwired: 2 in, 2 out]
  n324 = property on="Test Ring" class="Ring (strict)"("Visible"=w34) -> ()  [unwired: 2 in, 2 out]
  n325 = property on="Rev/Fwd" class="Clust (strict)"("Visible"=w34) -> ()  [unwired: 2 in, 2 out]
  n326 = while {
    tunnel: u16 1741 ("timeout ms (25000)") -> [w499]
    stop <- FALSE stop-if-true
    n327 = TCP Create Listener(10:w499) -> (0:w498:errorcluster, 3:w500:refnum<k5>)  [unwired: 4 in, 1 out]
    n328 = case shown="No Error" w498 {
      selector: w498 -> [w502 _]
      tunnel: w500 -> [w503 _]
      frame No Error {
        n329 = while {
          tunnel: w503 -> [w506]
          tunnel: w502 -> [w505]
          stop <- FALSE stop-if-true
          n330 = TCP Wait On Listener(8:w505, 11:w506) -> (0:w507:errorcluster, 4:w508:refnum<k5>)  [unwired: 2 in, 3 out]
          n331 = local write "TCP"(w508) -> ()
          n332 = case shown="No Error" w507 {
            frame No Error {
            }
            frame Error {
              n333 = Wait (ms)(milliseconds to wait=u32 1000) -> ()  [unwired: 1 out]
            }
          }
        }
      }
      frame Error {
        n334 = Wait (ms)(milliseconds to wait=u32 1000) -> ()  [unwired: 1 out]
      }
    }
  }
  n335 = local write "Command Selection"(u16 0 ("milliseconds to wait")) -> ()
  n336 = local write "Command Params"(string[][] [] ("Command Params")) -> ()
  n337 = global write "WPI_DashboardLogging Global.vi" "Recording"(w57) -> ()
  n338 = local write "Rec Mode"(w57) -> ()
  n339 = call <vilib>:"NT Write String.vi"("String"="Select Auto", "Name"="Auto Selector") -> ()  [unwired: 9 in, 1 out]
